vi "Digital Serial Acq Cfg Popup.vi"(8 "error in (no error)":errorcluster, 11 "config file in":path caption="Configuration File") -> (0 "error out":errorcluster, 2 "digital serial input settings":T2={"number of channels"=0, "data justification"=enum."Left Justified", "endianness"=enum."LSB First", "channel length"=0, "bit depth"=0, "frame clock rate"=0.0, "bit clock edge sync"=enum."Falling", "master clock source"=enum."Internal", "master clock rate"=2.0, "Logic Level"=enum."3.3 V", "frame sync edge for channel 0"=enum."Rising", "Channel 0 Offset"=0}, 3 "config file out":path caption="Configuration File")   [LabVIEW 2021, in "Audio Popup UI.lvlib"]
uses:
  Audio Popup UI.lvlib
  <vilib>/PDM Acquisition Toolkit/shared/controls/PCM Data Justification.ctl
  <vilib>/PDM Acquisition Toolkit/shared/PDM Shared.lvlib
  <vilib>/PDM Acquisition Toolkit/shared/controls/PCM Bit Endianness.ctl
  <vilib>/PDM Acquisition Toolkit/shared/controls/Digital Edge.ctl
  <vilib>/PDM Acquisition Toolkit/host/Classes/Session/Controls/Logic Levels.ctl
  <vilib>/PDM Acquisition Toolkit/host/Classes/Session/DecoderSession.lvclass
  digital serial input settings/Digital Serial Input Settings.lvlib
  <vilib>/Utility/miscctls.llb/LVPointTypeDef.ctl
  controls/digital audio protocol/master clock source.ctl
  controls/digital serial input settings.ctl
panel:
  in  "master clock source":T1 caption="Master clock source"
  in  "channel 0 offset":u32=1
  in  "Save":bool
  in  "logic level":enum32{"3.3 V", "1.8 V", "1.2 V"}(ring) caption="Logic level"
  in  "master clock rate":dbl=12288000.0 caption="Master clock rate" format="%#_6pHz"
  out "Bit clock rate":dbl=3072000.0 format="%#_6pHz"
  in  "number of channels":u32=2 caption="Number of channels"
  in  "TDM":bool
  in  "RJ":bool
  in  "LJ":bool
  in  "I2S":bool
  in  "bit clock edge sync":enum32{"Rising", "Falling"}(ring)=enum."Falling" caption="Bit clock edge sync"
  in  "frame clock rate":dbl=48000.0 caption="Frame clock rate" format="%#_6pHz"
  in  "data justification":enum32{"Left Justified", "Right Justified"}(ring) caption="Data justification"
  in  "endianness":enum32{"MSB First", "LSB First"}(ring) caption="Endianness"
  in  "bit depth":u32=24 caption="Bit depth"
  in  "channel length":u32=32 caption="Channel length"
  in  "frame sync edge for channel 0":enum32{"Rising", "Falling"}(ring)=enum."Falling" caption="Frame sync edge for Channel 0"
  # "Audio Protocol"
  # "Clock Settings"
  # "Signal Level"
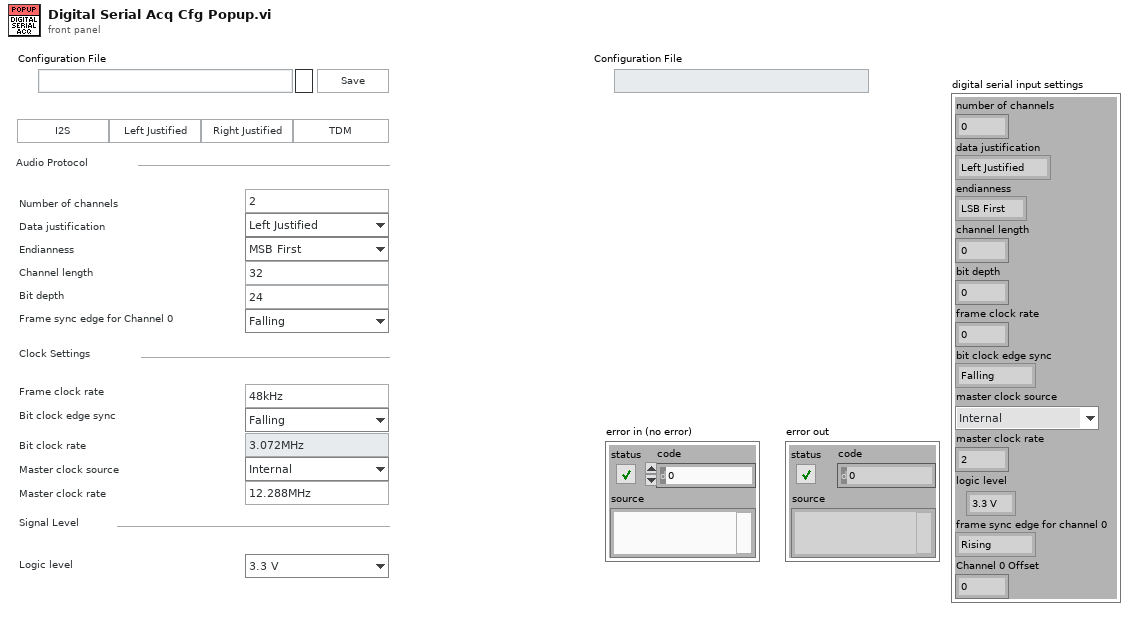
[diagram p1: front panel]
types:
  T1 = typedef "master clock source.ctl" = enum32{"Internal", "External"}
  T2 = typedef "digital serial input settings.ctl" = cluster{"number of channels":u32, "data justification":T3, "endianness":T4, "channel length":u32, "bit depth":u32, "frame clock rate":dbl, "bit clock edge sync":T5, "master clock source":T1, "master clock rate":dbl, "Logic Level":T6, "frame sync edge for channel 0":T5, "Channel 0 Offset":u32}
  T3 = typedef "PDM Shared.lvlib/PCM Data Justification.ctl" = enum16{"Left Justified", "Right Justified"}
  T4 = typedef "PDM Shared.lvlib/PCM Bit Endianness.ctl" = enum16{"MSB First", "LSB First"}
  T5 = typedef "PDM Shared.lvlib/Digital Edge.ctl" = enum8{"Rising", "Falling"}
  T6 = typedef "PDM Acquisition Class Library.lvlib/DecoderSession.lvclass/Logic Levels.ctl" = enum16{"3.3 V", "1.8 V", "1.2 V"}
  T7 = typedef "LVPointTypeDef.ctl" = cluster{"Horizontal":i16, "Vertical":i16}
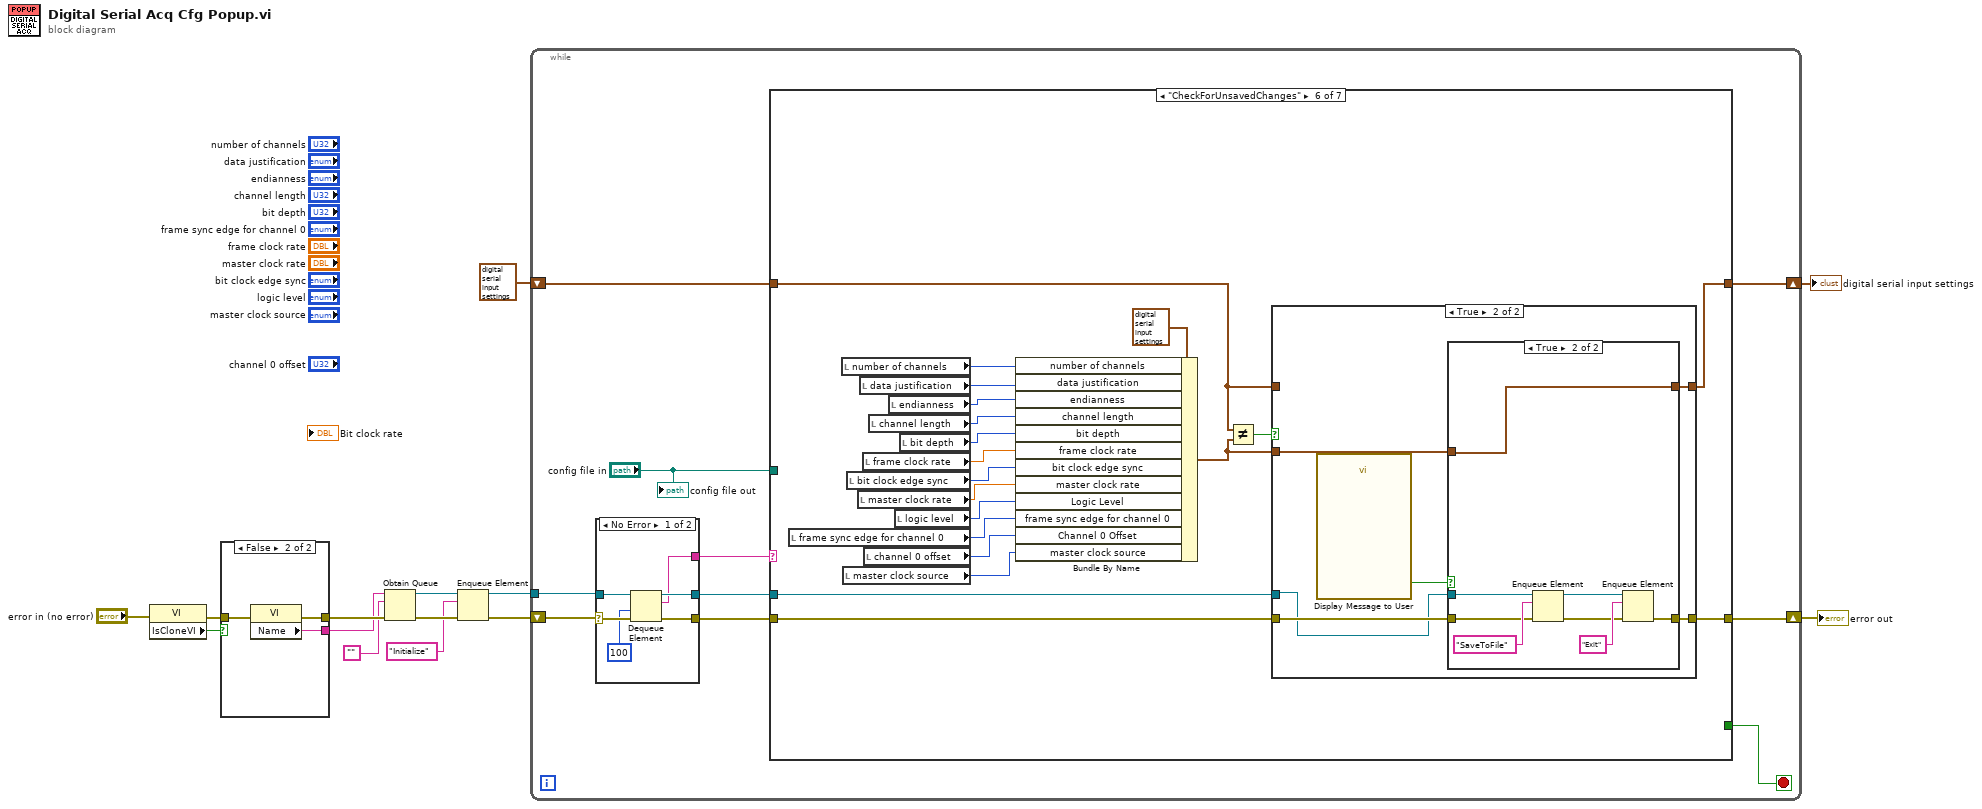
[diagram p0: block diagram]
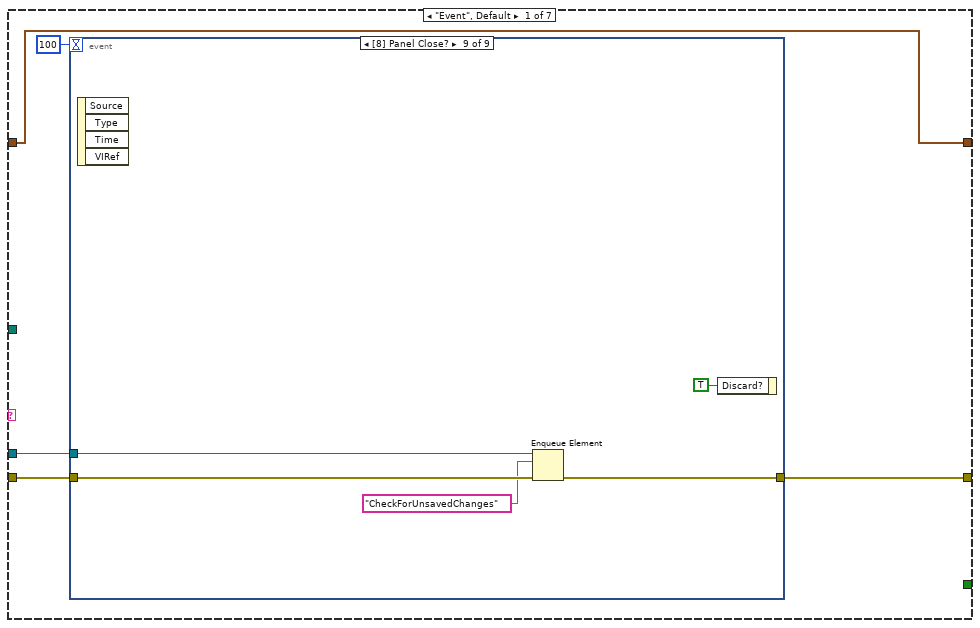
[diagram p2: hidden frame]
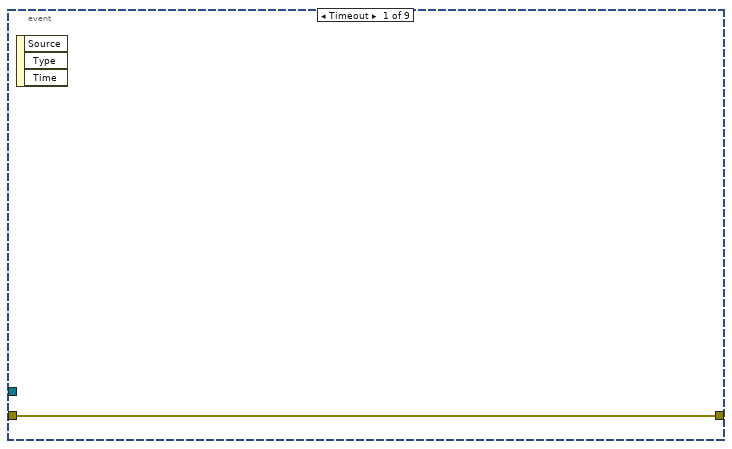
[diagram p3: hidden frame]
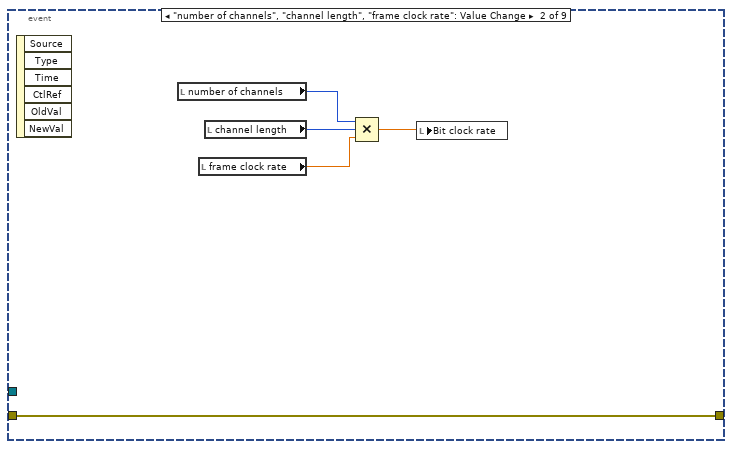
[diagram p4: hidden frame]
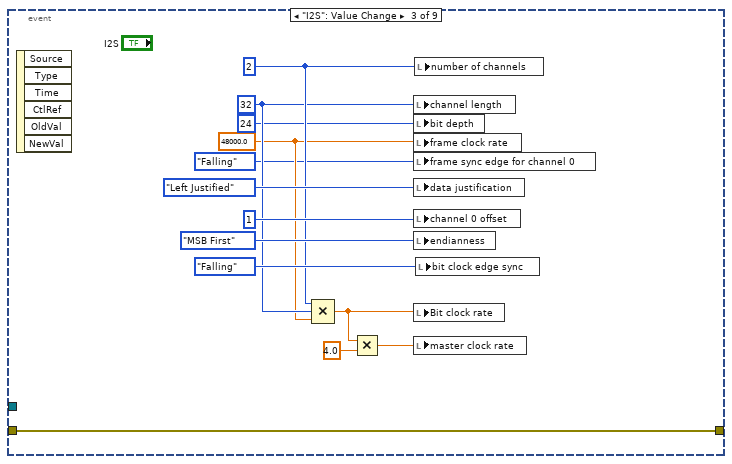
[diagram p5: hidden frame]
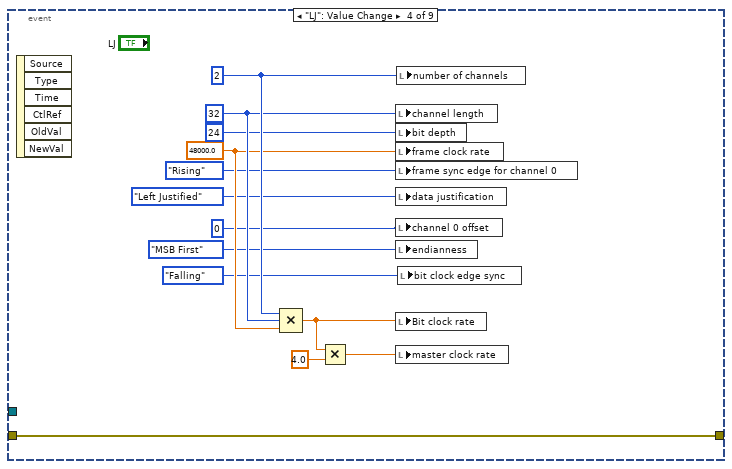
[diagram p6: hidden frame]
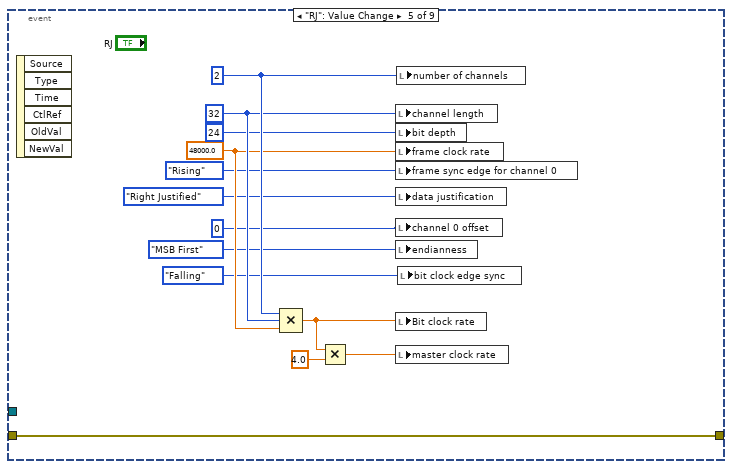
[diagram p7: hidden frame]
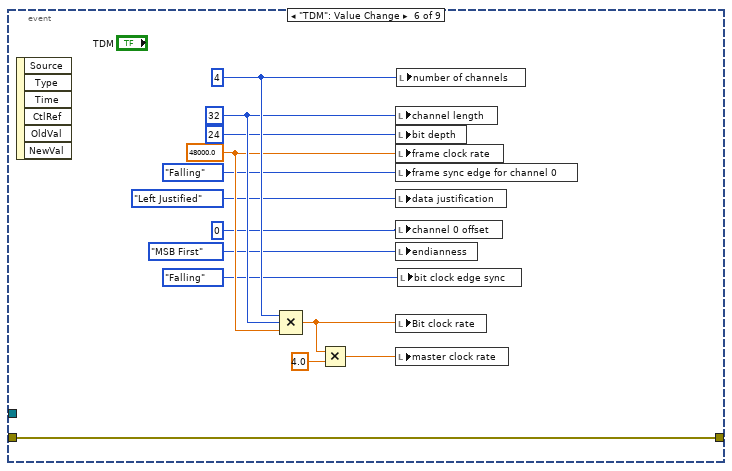
[diagram p8: hidden frame]
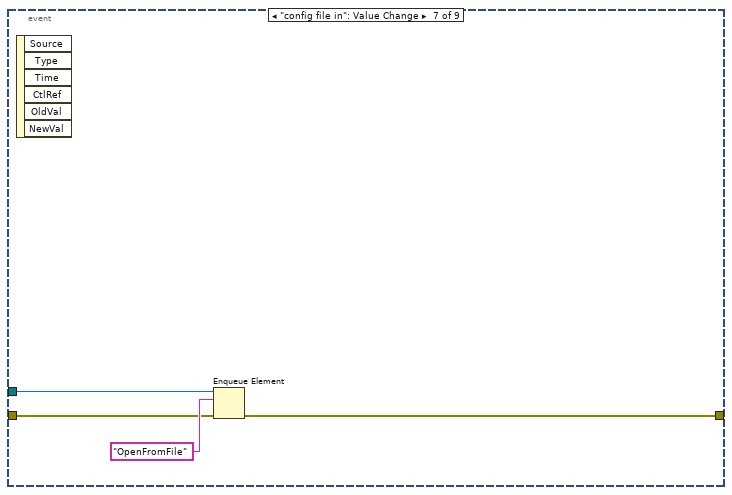
[diagram p9: hidden frame]
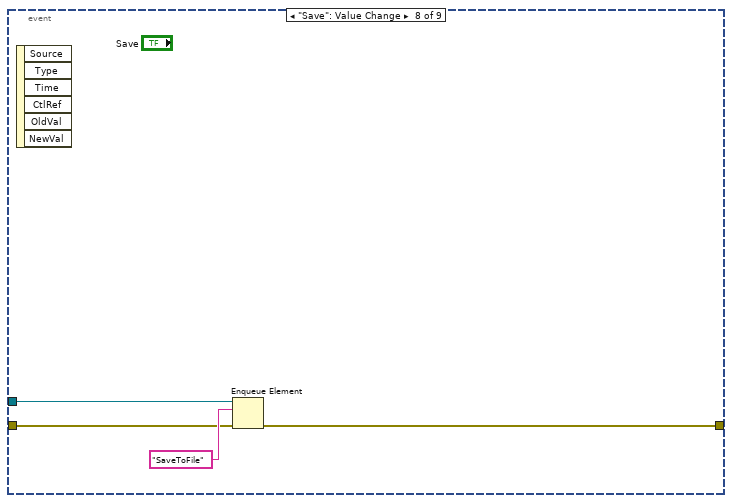
[diagram p10: hidden frame]
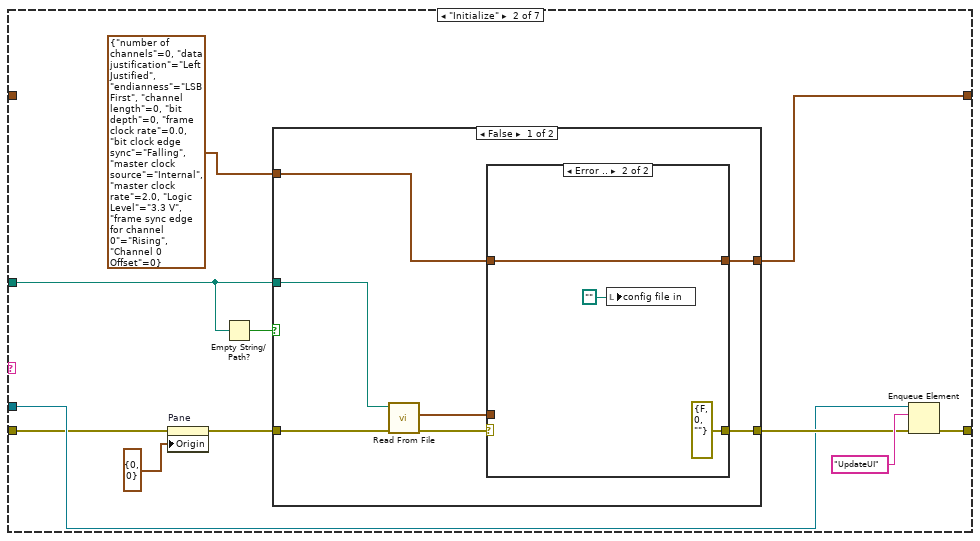
[diagram p11: hidden frame]
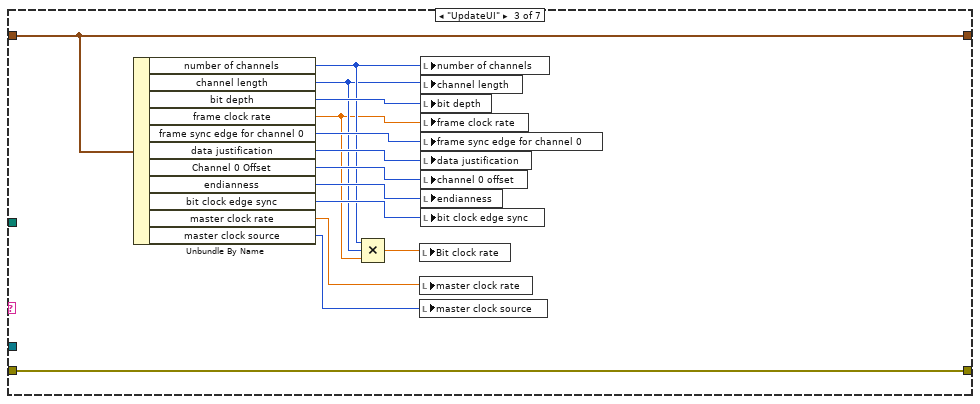
[diagram p14: hidden frame]
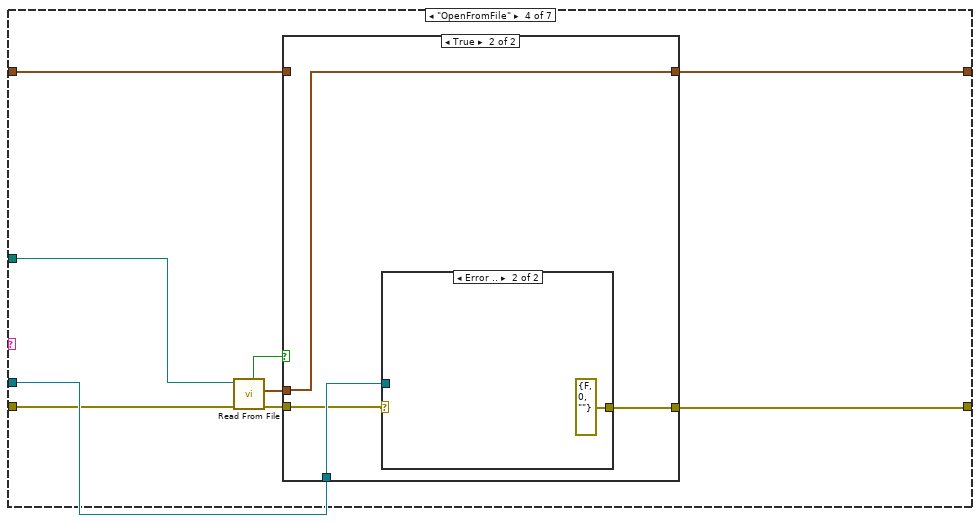
[diagram p15: hidden frame]
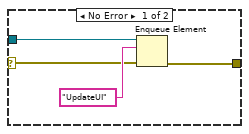
[diagram p17: hidden frame]
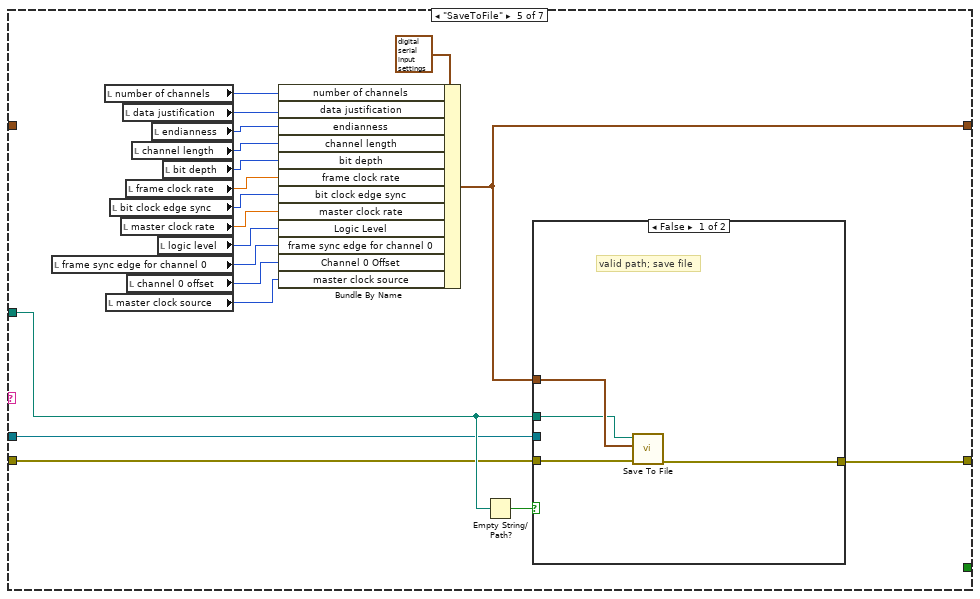
[diagram p18: hidden frame]
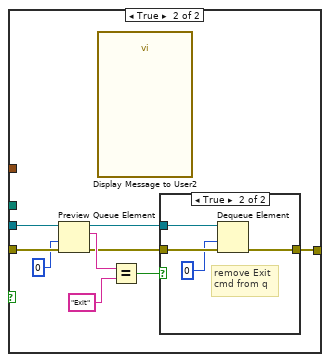
[diagram p19: hidden frame]
diagram:
  n1 = property class="VI"(error in="error in (no error)") -> (error out=w7:errorcluster, "IsCloneVI"=w8:bool)  [unwired: 1 in, 1 out]
  n2 = case shown="False" w8 {
    tunnel: [w17 w20] -> w14
    tunnel: [w16 w19] -> w13
    tunnel: w7 -> [w15 w18]
    frame True {
      n3 = property class="VI"(error in=w15) -> (error out=w17:errorcluster, "Clone Name"=w16:string)  [unwired: 1 in, 1 out]
    }
    frame False {
      n4 = property class="VI"(error in=w18) -> (error out=w20:errorcluster, "Name"=w19:string)  [unwired: 1 in, 1 out]
    }
  }
  n5 = Obtain Queue(name (unnamed)=w13, element data type="", error in (no error)=w14) -> (queue out=w11:refnum<queue>, error out=w12:errorcluster)  [unwired: 2 in, 1 out]
  n6 = Enqueue Element(queue=w11, element="Initialize", error in (no error)=w12) -> (queue out=w5:refnum<queue>, error out=w6:errorcluster)  [unwired: 1 in, 1 out]
  n7 = while {
    tunnel: w5 -> [w29]
    shift-right: [w25] -> w3
    shift-left: w6 -> [w30]
    shift-right: [w22] -> w1
    shift-left: T2 {"number of channels"=0, "data justification"=enum."Left Justified", "endianness"=enum."LSB First", "channel length"=0, "bit depth"=0, "frame clock rate"=0.0, "bit clock edge sync"=enum."Falling", "master clock source"=enum."Internal", "master clock rate"=2.0, "Logic Level"=enum."3.3 V", "frame sync edge for channel 0"=enum."Rising", "Channel 0 Offset"=0} ("digital serial input settings") -> [w23]
    stop <- w24 stop-if-true
    n8 = case shown="No Error" w30 {
      selector: w30 -> [w259 w262]
      tunnel: [w258 w262] -> w26
      tunnel: w29 -> [w257 w261]
      tunnel: [w256 w261] -> w27
      tunnel: [w255 "Handle Error"] -> w28
      frame No Error {
        n9 = Dequeue Element(queue=w257, timeout in ms (-1)=100, error in (no error)=w259) -> (queue out=w256:refnum<queue>, element=w255:string, error out=w258:errorcluster)  [unwired: 1 out]
      }
      frame Error {
      }
    }
    n10 = case shown="\"CheckForUnsavedChanges\"" w28 {
      tunnel: w27 -> [w33 w112 _ w154 w167 w206 w249]
      tunnel: w26 -> [w34 w110 w145 w151 w169 w209 w250]
      tunnel: [w32 w113 w145 w153 w172 w208 w247] -> w25
      tunnel: [_ _ _ _ _ _ TRUE] -> w24
      tunnel: w23 -> [w31 _ w144 w148 _ w204 w246]
      tunnel: [w31 w107 w144 w147 w171 w207 w246] -> w22
      tunnel: "config file in" -> [_ w116 _ w152 w170 _ _]
      frame "Event", Default {
        n11 = event shown="[8] Panel Close?" {
          selector: _ -> [_ _ _ _ _ _ _ _ _]
          dyn-events: _ -> [_ _ _ _ _ _ _ _ _]
          timeout: 100 -> [_ _ _ _ _ _ _ _ _]
          tunnel: w34 -> [w36 w37 w42 w55 w68 w81 w96 w100 w105]
          tunnel: w33 -> [_ _ _ _ _ _ w95 w99 w104]
          tunnel: [w36 w37 w42 w55 w68 w81 w94 w98 w103] -> w32
          event Timeout {
            n12 = event-data() -> ()  [unwired: 1 in, 3 out]
          }
          event "number of channels", "channel length", "frame clock rate": Value Change {
            n13 = event-data() -> ()  [unwired: 1 in, 6 out]
            n14 = local read "number of channels"() -> (w39:u32)
            n15 = local read "frame clock rate"() -> (w38:dbl)
            n16 = local read "channel length"() -> (w40:u32)
            n17 = Compound Arithmetic op=MULTIPLY(w39, w40, w38) -> (w41:dbl)
            n18 = local write "Bit clock rate"(w41) -> ()
          }
          event "I2S": Value Change {
            w45 = 48000.0 ("Frame Clock Rate")
            w46 = u32 32 ("Channel Length")
            w47 = u32 2 ("Number of Channels")
            n19 = event-data() -> ()  [unwired: 1 in, 6 out]
            n20 = Compound Arithmetic op=MULTIPLY(w47, w46, w45) -> (w53:dbl)
            n21 = Multiply(x=w53, y=4.0) -> (x*y=w52:dbl)
            n22 = local write "channel length"(w46) -> ()
            n23 = local write "bit depth"(u32 24 ("Bit Depth")) -> ()
            n24 = local write "frame clock rate"(w45) -> ()
            n25 = local write "frame sync edge for channel 0"(enum32{"Rising", "Falling"}."Falling" ("bit clock edge sync")) -> ()
            n26 = local write "data justification"(enum32{"Left Justified", "Right Justified"}."Left Justified" ("data justification")) -> ()
            n27 = local write "channel 0 offset"(u32 1 ("Channel 0 Offset")) -> ()
            n28 = local write "endianness"(enum32{"MSB First", "LSB First"}."MSB First" ("endianness")) -> ()
            n29 = local write "Bit clock rate"(w53) -> ()
            n30 = local write "master clock rate"(w52) -> ()
            n31 = local write "number of channels"(w47) -> ()
            n32 = local write "bit clock edge sync"(enum32{"Rising", "Falling"}."Falling" ("frame sync edge for channel 0")) -> ()
          }
          event "LJ": Value Change {
            w63 = 48000.0 ("Frame Clock Rate")
            w65 = u32 32 ("Channel Length")
            w66 = u32 2 ("Number of Channels")
            n33 = event-data() -> ()  [unwired: 1 in, 6 out]
            n34 = Compound Arithmetic op=MULTIPLY(w66, w65, w63) -> (w57:dbl)
            n35 = Multiply(x=w57, y=4.0) -> (x*y=w56:dbl)
            n36 = local write "channel length"(w65) -> ()
            n37 = local write "bit depth"(u32 24 ("Bit Depth")) -> ()
            n38 = local write "frame clock rate"(w63) -> ()
            n39 = local write "frame sync edge for channel 0"(enum32{"Rising", "Falling"}."Rising" ("bit clock edge sync")) -> ()
            n40 = local write "data justification"(enum32{"Left Justified", "Right Justified"}."Left Justified" ("data justification")) -> ()
            n41 = local write "channel 0 offset"(u32 0 ("Channel 0 Offset")) -> ()
            n42 = local write "endianness"(enum32{"MSB First", "LSB First"}."MSB First" ("endianness")) -> ()
            n43 = local write "Bit clock rate"(w57) -> ()
            n44 = local write "master clock rate"(w56) -> ()
            n45 = local write "number of channels"(w66) -> ()
            n46 = local write "bit clock edge sync"(enum32{"Rising", "Falling"}."Falling" ("frame sync edge for channel 0")) -> ()
          }
          event "RJ": Value Change {
            w76 = 48000.0 ("Frame Clock Rate")
            w78 = u32 32 ("Channel Length")
            w79 = u32 2 ("Number of Channels")
            n47 = event-data() -> ()  [unwired: 1 in, 6 out]
            n48 = Compound Arithmetic op=MULTIPLY(w79, w78, w76) -> (w70:dbl)
            n49 = Multiply(x=w70, y=4.0) -> (x*y=w69:dbl)
            n50 = local write "channel length"(w78) -> ()
            n51 = local write "bit depth"(u32 24 ("Bit Depth")) -> ()
            n52 = local write "frame clock rate"(w76) -> ()
            n53 = local write "frame sync edge for channel 0"(enum32{"Rising", "Falling"}."Rising" ("bit clock edge sync")) -> ()
            n54 = local write "data justification"(enum32{"Left Justified", "Right Justified"}."Right Justified" ("data justification")) -> ()
            n55 = local write "channel 0 offset"(u32 0 ("Channel 0 Offset")) -> ()
            n56 = local write "endianness"(enum32{"MSB First", "LSB First"}."MSB First" ("endianness")) -> ()
            n57 = local write "Bit clock rate"(w70) -> ()
            n58 = local write "master clock rate"(w69) -> ()
            n59 = local write "number of channels"(w79) -> ()
            n60 = local write "bit clock edge sync"(enum32{"Rising", "Falling"}."Falling" ("frame sync edge for channel 0")) -> ()
          }
          event "TDM": Value Change {
            w89 = 48000.0 ("Frame Clock Rate")
            w91 = u32 32 ("Channel Length")
            w92 = u32 4 ("Number of Channels")
            n61 = event-data() -> ()  [unwired: 1 in, 6 out]
            n62 = Compound Arithmetic op=MULTIPLY(w92, w91, w89) -> (w83:dbl)
            n63 = Multiply(x=w83, y=4.0) -> (x*y=w82:dbl)
            n64 = local write "channel length"(w91) -> ()
            n65 = local write "bit depth"(u32 24 ("Bit Depth")) -> ()
            n66 = local write "frame clock rate"(w89) -> ()
            n67 = local write "frame sync edge for channel 0"(enum32{"Rising", "Falling"}."Falling" ("bit clock edge sync")) -> ()
            n68 = local write "data justification"(enum32{"Left Justified", "Right Justified"}."Left Justified" ("data justification")) -> ()
            n69 = local write "channel 0 offset"(u32 0 ("Channel 0 Offset")) -> ()
            n70 = local write "endianness"(enum32{"MSB First", "LSB First"}."MSB First" ("endianness")) -> ()
            n71 = local write "Bit clock rate"(w83) -> ()
            n72 = local write "master clock rate"(w82) -> ()
            n73 = local write "number of channels"(w92) -> ()
            n74 = local write "bit clock edge sync"(enum32{"Rising", "Falling"}."Falling" ("frame sync edge for channel 0")) -> ()
          }
          event "config file in": Value Change {
            n75 = event-data() -> ()  [unwired: 1 in, 6 out]
            n76 = Enqueue Element(queue=w95, element="OpenFromFile", error in (no error)=w96) -> (error out=w94:errorcluster)  [unwired: 1 in, 2 out]
          }
          event "Save": Value Change {
            n77 = event-data() -> ()  [unwired: 1 in, 6 out]
            n78 = Enqueue Element(queue=w99, element="SaveToFile", error in (no error)=w100) -> (error out=w98:errorcluster)  [unwired: 1 in, 2 out]
          }
          event Panel Close? {
            n79 = event-data() -> ()  [unwired: 1 in, 4 out]
            n80 = Enqueue Element(queue=w104, element="CheckForUnsavedChanges", error in (no error)=w105) -> (error out=w103:errorcluster)  [unwired: 1 in, 2 out]
            n81 = event-data("Discard?"=TRUE) -> ()  [unwired: 1 in, 1 out]
          }
        }
      }
      frame "Initialize" {
        n82 = property on="Pane" class="Pane"(error in=w110, "Origin"=T7 {"Horizontal"=0, "Vertical"=0}) -> (error out=w109:errorcluster)  [unwired: 1 in, 1 out]
        n83 = Empty String/Path?(string/path=w116) -> (empty?=w117:bool)
        n84 = case shown="False" w117 {
          tunnel: w109 -> [w124 w131]
          tunnel: w116 -> [w123 _]
          tunnel: [w119 w130] -> w107
          tunnel: [w121 w131] -> w114
          tunnel: T2 {"number of channels"=0, "data justification"=enum."Left Justified", "endianness"=enum."LSB First", "channel length"=0, "bit depth"=0, "frame clock rate"=0.0, "bit clock edge sync"=enum."Falling", "master clock source"=enum."Internal", "master clock rate"=2.0, "Logic Level"=enum."3.3 V", "frame sync edge for channel 0"=enum."Rising", "Channel 0 Offset"=0} ("digital serial input settings") -> [w118 w130]
          frame False {
            n85 = call "Read From File.vi"("error in (no error)"=w124, "file path"=w123) -> ("error out"=w122:errorcluster, "digital serial input settings"=w120:T2)  [unwired: 7 in, 1 out]
            n86 = case shown="Error .." w122 {
              selector: w122 -> [w126 _]
              tunnel: [w126 errorcluster {"status"=FALSE, "code"=0, "source"=""} ("error IO")] -> w121
              tunnel: w120 -> [w125 _]
              tunnel: [w125 w129] -> w119
              tunnel: w118 -> [_ w129]
              frame No Error {
              }
              frame Error {
                n87 = local write "config file in"(path "") -> ()
              }
            }
          }
          frame True {
          }
        }
        n88 = Enqueue Element(queue=w112, element="UpdateUI", error in (no error)=w114) -> (error out=w113:errorcluster)  [unwired: 1 in, 2 out]
      }
      frame "UpdateUI" {
        n89 = Unbundle By Name(w144) -> ("number of channels"=w137:u32, "channel length"=w136:u32, "bit depth"=w143:u32, "frame clock rate"=w135:dbl, "frame sync edge for channel 0"=w142:T5, "data justification"=w141:T3, "Channel 0 Offset"=w140:u32, "endianness"=w139:T4, "bit clock edge sync"=w138:T5, "master clock rate"=w133:dbl, "master clock source"=w132:T1)
        n90 = Compound Arithmetic op=MULTIPLY(w137, w136, w135) -> (w134:dbl)
        n91 = local write "Bit clock rate"(w134) -> ()
        n92 = local write "master clock rate"(w133) -> ()
        n93 = local write "master clock source"(w132) -> ()
        n94 = local write "number of channels"(w137) -> ()
        n95 = local write "channel length"(w136) -> ()
        n96 = local write "bit depth"(w143) -> ()
        n97 = local write "frame clock rate"(w135) -> ()
        n98 = local write "frame sync edge for channel 0"(w142) -> ()
        n99 = local write "data justification"(w141) -> ()
        n100 = local write "channel 0 offset"(w140) -> ()
        n101 = local write "endianness"(w139) -> ()
        n102 = local write "bit clock edge sync"(w138) -> ()
      }
      frame "OpenFromFile" {
        n103 = call "Read From File.vi"("error in (no error)"=w151, "file path"=w152) -> ("error out"=w150:errorcluster, "digital serial input settings"=w146:T2, "file exists?"=w149:bool)  [unwired: 7 in]
        n104 = case shown="True" w149 {
          tunnel: w154 -> [_ w160]
          tunnel: [w155 w159] -> w153
          tunnel: w150 -> [w155 w157]
          tunnel: w148 -> [w156 _]
          tunnel: [w156 w158] -> w147
          tunnel: w146 -> [_ w158]
          frame False {
          }
          frame True {
            n105 = case shown="Error .." w157 {
              selector: w157 -> [w161 _]
              tunnel: w160 -> [w163 _]
              tunnel: [w162 errorcluster {"status"=FALSE, "code"=0, "source"=""} ("error out")] -> w159
              frame No Error {
                n106 = Enqueue Element(queue=w163, element="UpdateUI", error in (no error)=w161) -> (error out=w162:errorcluster)  [unwired: 1 in, 2 out]
              }
              frame Error {
              }
            }
          }
        }
      }
      frame "SaveToFile" {
        n107 = local read "frame sync edge for channel 0"() -> (w174:enum32{"Rising", "Falling"})
        n108 = local read "number of channels"() -> (w183:u32)
        n109 = local read "master clock source"() -> (w166:T1)
        n110 = local read "bit clock edge sync"() -> (w177:enum32{"Rising", "Falling"})
        n111 = local read "master clock rate"() -> (w176:dbl)
        n112 = local read "data justification"() -> (w182:enum32{"Left Justified", "Right Justified"})
        n113 = local read "frame clock rate"() -> (w178:dbl)
        n114 = local read "channel 0 offset"() -> (w173:u32)
        n115 = local read "channel length"() -> (w180:u32)
        n116 = local read "endianness"() -> (w181:enum32{"MSB First", "LSB First"})
        n117 = local read "logic level"() -> (w175:enum32{"3.3 V", "1.8 V", "1.2 V"})
        n118 = local read "bit depth"() -> (w179:u32)
        n119 = Bundle By Name(cluster=T2 {"number of channels"=0, "data justification"=enum."Left Justified", "endianness"=enum."LSB First", "channel length"=0, "bit depth"=0, "frame clock rate"=0.0, "bit clock edge sync"=enum."Falling", "master clock source"=enum."Internal", "master clock rate"=2.0, "Logic Level"=enum."3.3 V", "frame sync edge for channel 0"=enum."Rising", "Channel 0 Offset"=0} ("input cluster"), "number of channels"=w183, "data justification"=w182, "endianness"=w181, "channel length"=w180, "bit depth"=w179, "frame clock rate"=w178, "bit clock edge sync"=w177, "master clock rate"=w176, "Logic Level"=w175, "frame sync edge for channel 0"=w174, "Channel 0 Offset"=w173, "master clock source"=w166) -> (w171:T2)
        n120 = Empty String/Path?(string/path=w170) -> (empty?=w168:bool)
        n121 = case shown="False" w168 {
          tunnel: [w188 w190] -> w172
          tunnel: w171 -> [w187 _]
          tunnel: w170 -> [w186 _]
          tunnel: w169 -> [w185 w197]
          tunnel: w167 -> [_ w196]
          frame False {
            # "valid path; save file"
            n122 = call "Save To File.vi"("error in (no error)"=w185, "digital serial input settings"=w187, "file path"=w186) -> ("error out"=w188:errorcluster)  [unwired: 8 in]
          }
          frame True {
            n123 = Preview Queue Element(queue=w196, timeout in ms (-1)=0, error in (no error)=w197) -> (queue out=w193:refnum<queue>, element=w195:string, error out=w191:errorcluster)  [unwired: 1 out]
            n124 = call "Display Message to User2"() -> ()  [unwired: 10 in, 2 out]
            n125 = Equal?(x=w195, y="Exit") -> (x = y?=w192:bool)
            n126 = case shown="True" w192 {
              tunnel: w193 -> [_ w202]
              tunnel: w191 -> [w198 w201]
              tunnel: [w198 w200] -> w190
              frame False {
              }
              frame True {
                # "remove Exit\ncmd from q"
                n127 = Dequeue Element(queue=w202, timeout in ms (-1)=0, error in (no error)=w201) -> (error out=w200:errorcluster)  [unwired: 3 out]
              }
            }
          }
        }
      }
      frame "CheckForUnsavedChanges" {
        n128 = local read "frame sync edge for channel 0"() -> (w213:enum32{"Rising", "Falling"})
        n129 = local read "number of channels"() -> (w222:u32)
        n130 = local read "master clock source"() -> (w203:T1)
        n131 = local read "bit clock edge sync"() -> (w216:enum32{"Rising", "Falling"})
        n132 = local read "master clock rate"() -> (w215:dbl)
        n133 = local read "data justification"() -> (w221:enum32{"Left Justified", "Right Justified"})
        n134 = local read "frame clock rate"() -> (w217:dbl)
        n135 = local read "channel 0 offset"() -> (w212:u32)
        n136 = local read "channel length"() -> (w219:u32)
        n137 = local read "endianness"() -> (w220:enum32{"MSB First", "LSB First"})
        n138 = local read "logic level"() -> (w214:enum32{"3.3 V", "1.8 V", "1.2 V"})
        n139 = local read "bit depth"() -> (w218:u32)
        n140 = Bundle By Name(cluster=T2 {"number of channels"=0, "data justification"=enum."Left Justified", "endianness"=enum."LSB First", "channel length"=0, "bit depth"=0, "frame clock rate"=0.0, "bit clock edge sync"=enum."Falling", "master clock source"=enum."Internal", "master clock rate"=2.0, "Logic Level"=enum."3.3 V", "frame sync edge for channel 0"=enum."Rising", "Channel 0 Offset"=0} ("input cluster"), "number of channels"=w222, "data justification"=w221, "endianness"=w220, "channel length"=w219, "bit depth"=w218, "frame clock rate"=w217, "bit clock edge sync"=w216, "master clock rate"=w215, "Logic Level"=w214, "frame sync edge for channel 0"=w213, "Channel 0 Offset"=w212, "master clock source"=w203) -> (w205:T2)
        n141 = Not Equal?(x=w204, y=w205) -> (x != y?=w210:bool)
        n142 = case shown="True" w210 {
          tunnel: w209 -> [w225 w233]
          tunnel: [w223 w229] -> w208
          tunnel: w205 -> [_ w231]
          tunnel: w204 -> [w227 _]
          tunnel: [w227 w230] -> w207
          tunnel: w206 -> [w224 w228]
          frame False {
            n143 = Enqueue Element(queue=w224, element="Exit", error in (no error)=w225) -> (error out=w223:errorcluster)  [unwired: 1 in, 2 out]
          }
          frame True {
            n144 = call "Display Message to User"() -> ("Yes"=w232:bool)  [unwired: 10 in, 1 out]
            n145 = case shown="True" w232 {
              tunnel: w233 -> [w237 w244]
              tunnel: w231 -> [_ w243]
              tunnel: [_ w243] -> w230
              tunnel: [w235 w239] -> w229
              tunnel: w228 -> [w236 w238]
              frame False {
                n146 = Enqueue Element(queue=w236, element="Exit", error in (no error)=w237) -> (error out=w235:errorcluster)  [unwired: 1 in, 2 out]
              }
              frame True {
                n147 = Enqueue Element(queue=w238, element="SaveToFile", error in (no error)=w244) -> (queue out=w240:refnum<queue>, error out=w241:errorcluster)  [unwired: 1 in, 1 out]
                n148 = Enqueue Element(queue=w240, element="Exit", error in (no error)=w241) -> (error out=w239:errorcluster)  [unwired: 1 in, 2 out]
              }
            }
          }
        }
      }
      frame "Exit" {
        n149 = Flush Queue(queue=w249, error in (no error)=w250) -> (queue out=w253:refnum<queue>, error out=w252:errorcluster)  [unwired: 1 out]
        n150 = Release Queue(queue=w253, force destroy? (F)=TRUE, error in (no error)=w252) -> (error out=w247:errorcluster)  [unwired: 2 out]
      }
    }
    "config file out" <- "config file in"
  }
  "error out" <- w3
  "digital serial input settings" <- w1
